vi "MAIN game.vi"() -> ()   [LabVIEW 2018]
doc: "This program is a simple implementation of the classic game Pong. The user interface consists of an array of LEDs and a keyboard to control the position of the paddle. sThe game works on main principle that the ball has four attributes, x position, y position, x velocity and y velocity."
uses:
  right or left wall.ctl
  <vilib>/Utility/inputDevices.llb/keyboardAcquire.vi
  <vilib>/Utility/inputDevices.llb/closeKeyboard.vi
panel:
  out "Array":bool[][](array[boolean])
  out "Gracz 1 Wynik":i32
  out "Gracz 2 Wynik":i32
  in  "Loop Rate":u32=50
  in  "stop":bool
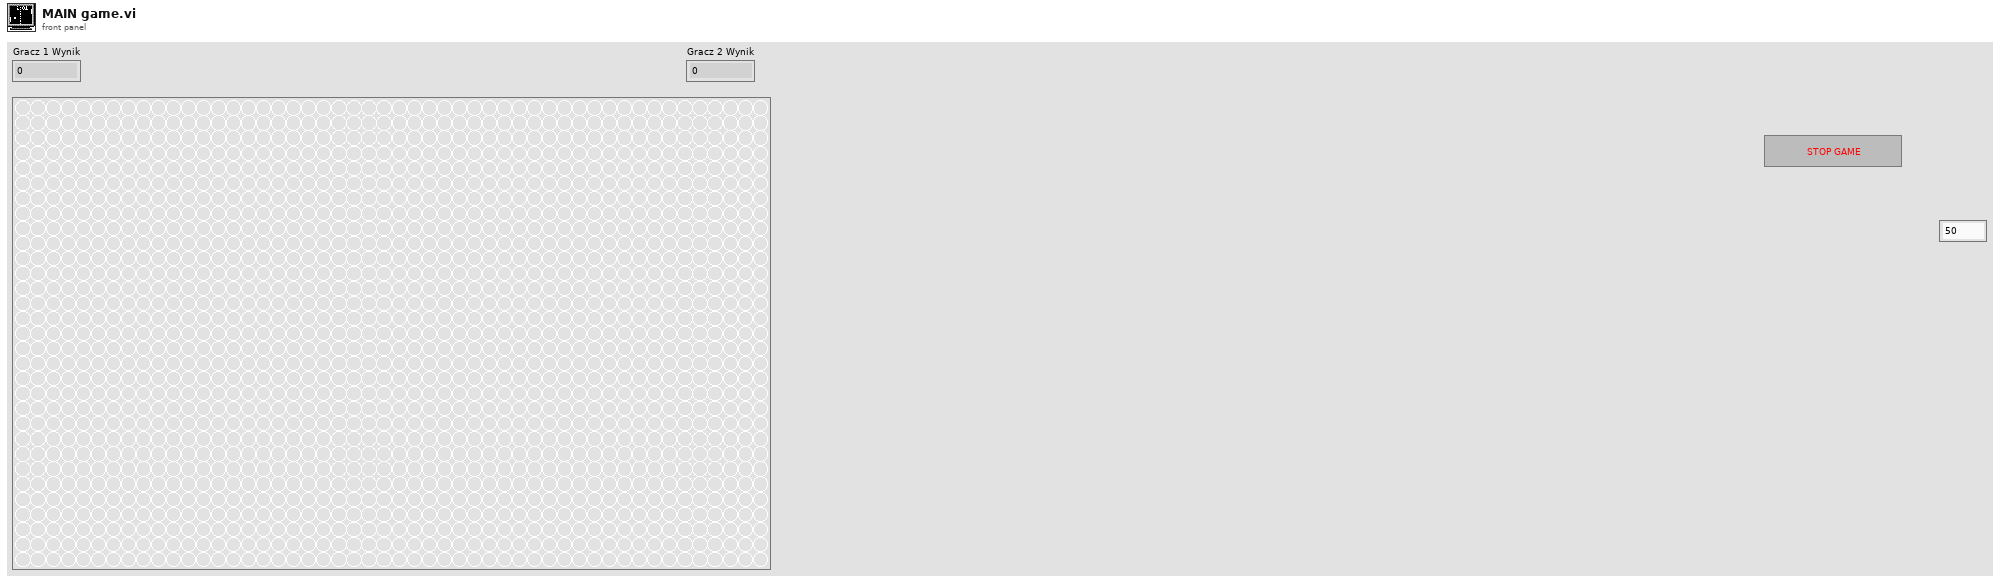
[diagram p1: front panel]
types:
  T1 = typedef "right or left wall.ctl" = enum16{"Left Wall", "Right Wall"}
  T2 = enum16{"0", "1", "2", "3", "4", "5", "6", "7", "8", "9", "A", "B", "C", "D", "E", "F", "G", "H", "I", "J", "K", "L", "M", "N", "O", "P", "Q", "R", "S", "T", "U", "V", "W", "X", "Y", "Z", "F1", "F2", "F3", "F4", "F5", "F6", "F7", "F8", "F9", "F10", "F11", "F12", "F13", "F14", "F15", "ADD", "BACK", "BACKSLASH", "CAPITAL", "COMMA", "DECIMAL", "DELETE", "DIVIDE", "DOWN", "END", "EQUALS", "ESCAPE", "GRAVE (`)", "HOME", "INSERT", "LBRACKET", "LCONTROL", "LEFT", "L ALT", "LSHIFT", "LWIN", "MINUS", "MULTIPLY", "NEXT", "NUMLOCK", "NUMPAD_0", "NUMPAD_1", "NUMPAD_2", "NUMPAD_3", "NUMPAD_4", "NUMPAD_5", "NUMPAD_6", "NUMPAD_7", "NUMPAD_8", "NUMPAD_9", "PAUSE", "PERIOD", "PRIOR (PG UP)", "RBRACKET", "RCONTROL", "RETURN", "RIGHT", "R ALT", "RSHIFT", "RWIN", "SCROLL", "SEMICOLON", "SLASH", "SPACE", "SUBTRACT", "TAB", "UP", "ENTER (num pad)", "' (quote)"}[]
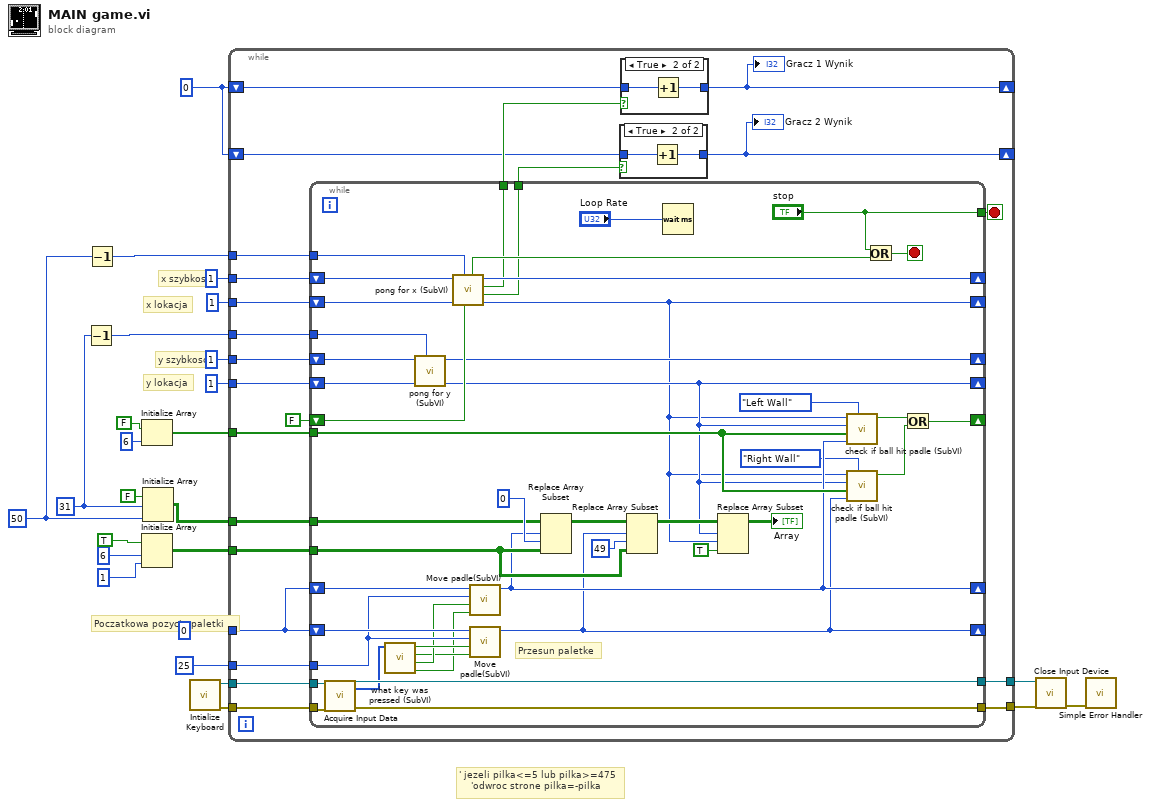
[diagram p0: block diagram]
diagram:
  w2 = 0
  w10 = 50 ("dimension size")
  w6 = 31 ("dimension size")
  # "y lokacja"
  # "y szybkosc"
  # "x lokacja"
  # "x szybkosc"
  # "' jezeli pilka<=5 lub pilka>=475\n    'odwroc strone pilka=-pilka"
  # "Poczatkowa pozycja paletki"
  n1 = Decrement(x=w6) -> (x-1=w9:i32)
  n2 = Decrement(x=w10) -> (x-1=w11:i32)
  n3 = Initialize Array(FALSE, 6 ("dimension size")) -> (w7:bool[])
  n4 = Initialize Array(TRUE ("stop"), 6 ("dimension size"), 1 ("dimension size")) -> (w16:bool[][])
  n5 = Initialize Array(FALSE, w6, w10) -> (w20:bool[][])
  n6 = call <vilib>:"Intialize Keyboard.vi"() -> ("error out"=w18:errorcluster, "device ID"=w19:refnum<k1>)  [unwired: 10 in]
  n7 = while {
    tunnel: 1 -> [w48]
    tunnel: 1 ("yLocation") -> [w47]
    tunnel: 1 ("ySpeed") -> [w46]
    tunnel: 1 ("xSpeed") -> [w45]
    tunnel: w20 -> [w44]
    tunnel: w19 -> [w43]
    tunnel: w18 -> [w42]
    tunnel: w16 -> [w41]
    tunnel: [w40] -> w15
    tunnel: [w26] -> w14
    tunnel: w11 -> [w39]
    tunnel: w9 -> [w38]
    tunnel: w7 -> [w37]
    tunnel: 0 -> [w36]
    tunnel: 25 -> [w35]
    shift-right: [w32] -> _
    shift-left: w2 -> [w33]
    shift-right: [w31] -> _
    shift-left: w2 -> [w30]
    stop <- w28 stop-if-true
    n8 = while {
      tunnel: w44 -> [w95]
      shift-right: [w63] -> _
      shift-left: w48 -> [w64]
      shift-right: [w72] -> _
      shift-left: w47 -> [w78]
      tunnel: w39 -> [w66]
      shift-right: [w73] -> _
      shift-left: w46 -> [w77]
      shift-right: [w62] -> _
      shift-left: w45 -> [w65]
      tunnel: w43 -> [w98]
      tunnel: w42 -> [w55]
      shift-right: [w74] -> _
      shift-left: w36 -> [w93]
      tunnel: w41 -> [w90]
      tunnel: [w97] -> w40
      tunnel: [w56] -> w26
      tunnel: w38 -> [w76]
      shift-right: [w69] -> _
      shift-left: FALSE -> [w79]
      tunnel: w37 -> [w82]
      tunnel: w35 -> [w86]
      shift-right: [w75] -> _
      shift-left: w36 -> [w87]
      tunnel: [w60] -> w34
      tunnel: [w59] -> w29
      tunnel: ["stop"] -> w28
      stop <- w68 stop-if-true
      # "Przesun paletke"
      n9 = call-poly <vilib>:"Acquire Input Data.vi"("device ID"=w98, "error in (no error)"=w55) -> ("device ID"=w97:refnum<k1>, "keys pressed"=w91:T2, "error out"=w56:errorcluster)  [unwired: 15 in]
      n10 = call "what key was pressed (SubVI).vi"("keys pressed"=w91) -> ("D"=w83:bool, "A"=w85:bool, "Left"=w84:bool, "Right"=w92:bool)  [unwired: 7 in]
      n11 = call "pong for y (SubVI).vi"("Numeric in"=w76, "y"=w78, "y szybkosc"=w77) -> ("Numeric out"=w72:i32, "y szybkosc wyjsciowa"=w73:i32)  [unwired: 7 in]
      n12 = call "pong for x (SubVI).vi"("Pilka uderzyla w paletke"=w79, "Numeric in"=w66, "loakcja x"=w64, "szybkosc x"=w65) -> ("lokacja x wyjsciowa"=w63:i32, "Pilka uderzyla w lewa sciane"=w59:bool, "Pilka uderzyla w prawa sciane"=w60:bool, "szybkosc x wyjsciowa"=w62:i32, "Pilka uderzyla w prawa lub lewa sicane"=w61:bool)  [unwired: 3 in]
      n13 = call "Move padle(SubVI).vi"("Lewy"=w83, "Prawy"=w85, "Max długości pola paletki"=w86, "Obecna pozycja paletki"=w87) -> ("Nowa pozycja paletki"=w75:i32)  [unwired: 7 in]
      n14 = call "Move padle(SubVI).vi"("Lewy"=w84, "Prawy"=w92, "Max długości pola paletki"=w86, "Obecna pozycja paletki"=w93) -> ("Nowa pozycja paletki"=w74:i32)  [unwired: 7 in]
      n15 = Replace Array Subset(array=w95, new element=w90, index (row)=w75, index (col)=0 ("disabled index (col)")) -> (w89:bool[][])
      n16 = Replace Array Subset(array=w89, new element=w90, index (row)=w74, index (col)=49) -> (w88:bool[][])
      n17 = Wait (ms)(milliseconds to wait="Loop Rate") -> ()  [unwired: 1 out]
      n18 = Replace Array Subset(array=w88, new element=TRUE ("new element/subarray"), index (row)=w72, index (col)=w63) -> (→"Array":bool[][])
      n19 = call "check if ball hit padle (SubVI).vi"(7:right_or_left_wall."Left Wall", "Nowa pozycja paletki"=w75, "Array"=w82, "lokacja y"=w72, "lokacja x"=w63) -> ("Czy pilka uderzyla w paletke?"=w80:bool)  [unwired: 6 in]
      n20 = call "check if ball hit padle (SubVI).vi"(7:right_or_left_wall."Right Wall", "Nowa pozycja paletki"=w74, "Array"=w82, "lokacja y"=w72, "lokacja x"=w63) -> ("Czy pilka uderzyla w paletke?"=w81:bool)  [unwired: 6 in]
      n21 = Or(x="stop", y=w61) -> (x .or. y?=w68:bool)
      n22 = Or(x=w80, y=w81) -> (x .or. y?=w69:bool)
    }
    n23 = case shown="True" w29 {
      tunnel: [w49 w51] -> w31
      tunnel: w30 -> [w49 w50]
      frame False {
      }
      frame True {
        n24 = Increment(x=w50) -> (x+1=w51:i32)
      }
    }
    "Gracz 2 Wynik" <- w31
    n25 = case shown="True" w34 {
      tunnel: [w52 w54] -> w32
      tunnel: w33 -> [w52 w53]
      frame False {
      }
      frame True {
        n26 = Increment(x=w53) -> (x+1=w54:i32)
      }
    }
    "Gracz 1 Wynik" <- w32
  }
  n27 = call-poly <vilib>:"Close Input Device.vi"("error in (no error)"=w14, "device ID"=w15) -> ("error out"=w1:errorcluster)  [unwired: 8 in]
  n28 = call <vilib>:"Simple Error Handler.vi"("error in (no error)"=w1) -> ()  [unwired: 4 in, 5 out]
